vi "Read Temp.vi"() -> (3 "temp":dbl caption="Temperature" format="%#_8g")   [LabVIEW 2009, in "Magnet.lvclass"]
uses:
  Magnet.lvclass
  Global/Temp Controller.vi
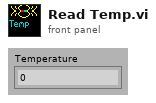
[diagram p1: front panel]
types:
  T1 = typedef "ITCIO.ctl" = cluster{"Address":T2, "Version":T3, "Ch 1 dec places":i16, "Ch 2 dec places":i16, "Ch 3 dec places":i16, "Ch1 Name":string, "Ch2 Name":string, "Ch3 Name":string}
  T2 = typedef "OxfordAddress.ctl" = cluster{"Com Port":i32, "ISOBUS Address":i32, "GPIB Address":i16, "Communication":enum16{"RS232", "ISOBUS", "GPIB", "Gateway"}}
  T3 = typedef "ITCVersion.ctl" = enum16{"ITC502", "ITC503", "ITC601"}
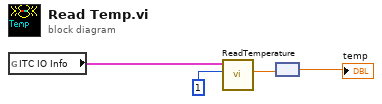
[diagram p0: block diagram]
diagram:
  n1 = global read "Temp Controller.vi" "ITC IO Info"() -> (w1:T1)
  n2 = call "ReadTemperature.vi"("Channel"=1, "IO Info"=w1) -> ("Temperature"=w3:dbl[unit])  [unwired: 5 out]
  n3 = node(w3) -> (→"temp":dbl)
